vi "as_state_driver.vi"(1 "AS_State":dbl) -> (0 "Name of state":string)   [LabVIEW 2017]
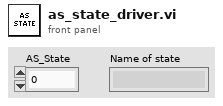
[diagram p1: front panel]
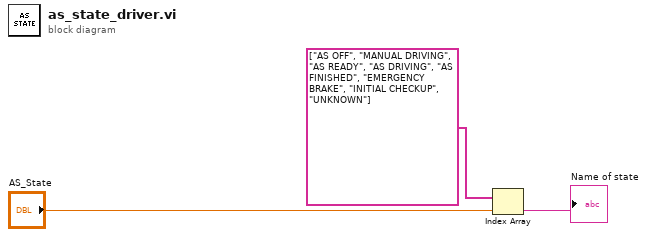
[diagram p0: block diagram]
diagram:
  n1 = Index Array(array=string[] ["AS OFF", "MANUAL DRIVING", "AS READY", "AS DRIVING", "AS FINISHED", "EMERGENCY BRAKE", "INITIAL CHECKUP", "UNKNOWN"], index="AS_State") -> (element=→"Name of state":string)
